vi "DSF.Shared.Configuration.Transfer.Get Channel Count.vi"(8 "error in (no error)":errorcluster, 11 "Transfer Configuration in":refnum<class "DSF.Shared.Configuration.Transfer.lvclass">) -> (0 "error out":errorcluster, 2 "channel count":u64, 3 "Transfer Configuration out":refnum<class "DSF.Shared.Configuration.Transfer.lvclass">)   [LabVIEW 2016, in "DSF.Shared.lvlib" / "DSF.Shared.Configuration.Transfer.lvclass"]
uses:
  DSF.Shared.Configuration.Transfer.lvclass
  DSF.Shared.Configuration.Transfer.lvclass/DSF.Shared.Configuration.Transfer.ctl
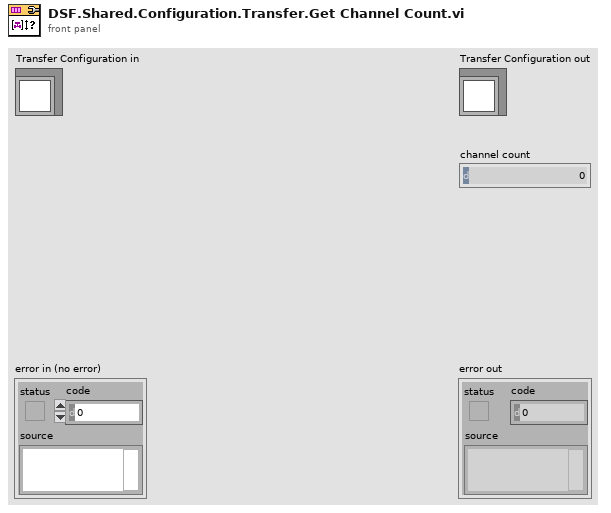
[diagram p1: front panel]
types:
  T1 = typedef "DSF.Shared.lvlib/DSF.Shared.Typedefs.Configuration.Transfer.Channel Descriptor.ctl" = cluster{"Channel Parameters":T2, "VS Channel Ref":T4}
  T2 = typedef "DSF.Shared.lvlib/DSF.Shared.Typedefs.Configuration.Transfer.Channel Parameters.ctl" = cluster{"offset":u64, "data type":T3}
  T3 = typedef "DSF.Shared.lvlib/DSF.Shared.Typedefs.Data Type.ctl" = enum8{"Bool", "SGL", "DBL", "I8", "I16", "I32", "I64", "U8", "U16", "U32", "U64"}
  T4 = typedef "Custom Device API.lvlib/Custom Device Item Ref.ctl" = u64
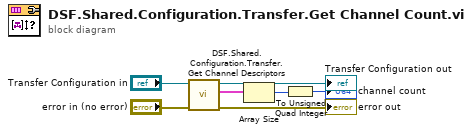
[diagram p0: block diagram]
diagram:
  n1 = call "DSF.Shared.Configuration.Transfer.Get Channel Descriptors.vi"("Transfer Configuration in"="Transfer Configuration in") -> ("Channel Descriptors"=w5:T1[], "Transfer Configuration out"=→"Transfer Configuration out":refnum<class "DSF.Shared.Configuration.Transfer.lvclass">)  [unwired: 9 in]
  n2 = Array Size(array=w5) -> (size(s)=w3:i32)
  n3 = To Unsigned Quad Integer(1:w3) -> (0:→"channel count":u64)
  "error out" <- "error in (no error)"
